vi "layout.vi"(0 "reference in":refnum<class "VINode.lvclass">, 1 "graph":refnum<class "Graph.lvclass">, 2 "graphics":refnum<class "Graphics.lvclass">, 3 "grid":refnum<class "Grid.lvclass">, 5 "error in (no error)":errorcluster) -> (14 "reference out":refnum<class "VINode.lvclass">, 19 "error out":errorcluster)   [LabVIEW 2020, in "VINode.lvclass"]
doc: "public void layout(Graph g, Graphics2D g2, Grid grid)"
uses:
  <resource>/Framework/Providers/Open_GDS/UML/VINode_class/VINode.lvclass
  C:/Program Files (x86)/National Instruments/LabVIEW 2020/resource/Framework/Providers/Open_GDS/UML/RectangularNode_class/RectangularNode.lvclass
  <resource>/Framework/Providers/Open_GDS/UML/Graph_class/Graph.lvclass
  <resource>/Framework/Providers/Open_GDS/UML/Graphics_class/Graphics.lvclass
  <resource>/Framework/Providers/Open_GDS/UML/Grid_class/Grid.lvclass
  <resource>/Framework/Providers/Open_GDS/UML/General/Rectangle/Rectangle Rectangle2D.ctl
  <resource>/Framework/Providers/Open_GDS/UML/MultiLineString_class/MultiLineString.lvclass
  <resource>/Framework/Providers/Open_GDS/UML/RectangularNode_class/RectangularNode.lvclass
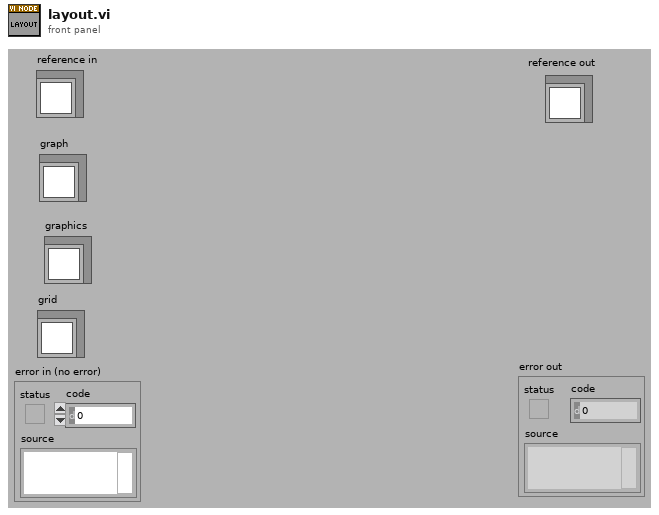
[diagram p1: front panel]
types:
  T1 = typedef "Rectangle Rectangle2D.ctl" = cluster{"x":dbl, "y":dbl, "width":dbl, "height":dbl}
  T2 = typedef "VINode.lvclass/ObjectAttributes.ctl" = cluster{"midHeight":dbl, "botHeight":dbl, "Name":refnum<class "MultiLineString.lvclass">, "DEFAULT_COMPARTMENT_HEIGHT":i32, "DEFAULT_WIDTH":i32, "DEFAULT_HEIGHT":i32, "VIPath":path, "Description":refnum<class "MultiLineString.lvclass">, "ShowDescription":bool}
  T3 = typedef "RectangularNode.lvclass/ObjectAttributes.ctl" = cluster{"bounds":T1}
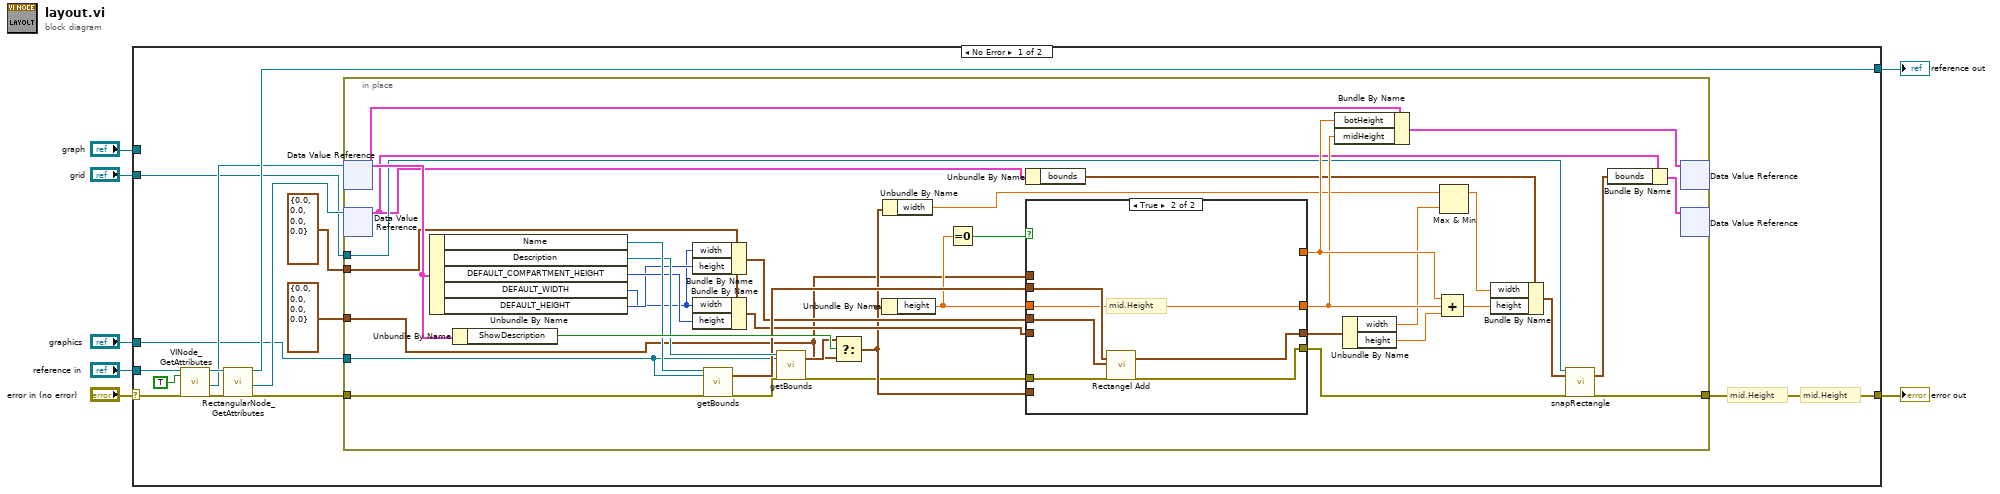
[diagram p0: block diagram]
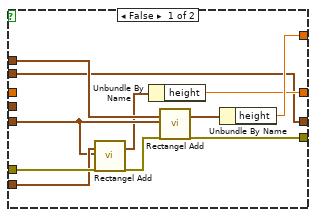
[diagram p2: hidden frame]
diagram:
  n1 = case shown="No Error" "error in (no error)" {
    selector: "error in (no error)" -> [w18 w76]
    tunnel: "reference in" -> [w21 w77]
    tunnel: [w20 w76] -> w6
    tunnel: [w19 w77] -> w5
    tunnel: "graph" -> [_ _]
    tunnel: "graphics" -> [w10 _]
    tunnel: "grid" -> [w8 _]
    frame No Error {
      # "mid.Height"
      # "mid.Height"
      n2 = call <resource>:"VINode_GetAttributes.vi"("reference in"=w21, "OnlyGetDvrReference(False)"=TRUE, "error in (no error)"=w18) -> ("reference out"=w16:refnum<class "VINode.lvclass">, "DataRef"=w14:refnum<data-value>, "error out"=w15:errorcluster)  [unwired: 13 in, 1 out]
      n3 = call <resource>:"RectangularNode_GetAttributes.vi"("reference in"=w16, "error in (no error)"=w15) -> ("reference out"=w19:refnum<class "VINode.lvclass">, "DataRef"=w13:refnum<data-value>, "error out"=w11:errorcluster)  [unwired: 14 in, 1 out]
      n4 = in-place {
        in-place-border: T1 {"x"=0.0, "y"=0.0, "width"=0.0, "height"=0.0} ("f") -> [w25]
        in-place-border: w11 -> [w39]
        in-place-border: w10 -> [w37]
        in-place-border: T1 {"x"=0.0, "y"=0.0, "width"=0.0, "height"=0.0} ("bounds") -> [w36]
        in-place-border: w8 -> [w35]
        in-place-border: [w32] -> w20
        n5 = in-place-dvr #1(w14) -> (w58:T2)  [unwired: 1 out]
        n6 = in-place-dvr #2(w13) -> (w28:T3)  [unwired: 1 out]
        n7 = Unbundle By Name(w58) -> ("Name"=w53:refnum<class "MultiLineString.lvclass">, "Description"=w52:refnum<class "MultiLineString.lvclass">, "DEFAULT_COMPARTMENT_HEIGHT"=w51:i32, "DEFAULT_WIDTH"=w22:i32, "DEFAULT_HEIGHT"=w50:i32)
        n8 = Unbundle By Name(w58) -> ("ShowDescription"=w54:bool)
        n9 = Bundle By Name(cluster=w36, "width"=w22, "height"=w50) -> (w48:T1)
        n10 = Bundle By Name(cluster=w36, "width"=w22, "height"=w51) -> (w47:T1)
        n11 = call-dynamic "getBounds.vi"("reference"=w53, "graphics"=w37, "error in (no error)"=w39) -> ("bounds"=w49:T1, "error out"=w38:errorcluster)  [unwired: 15 out]
        n12 = call-dynamic "getBounds.vi"("reference"=w52, "graphics"=w37, "error in (no error)"=w38) -> ("bounds"=w40:T1, "error out"=w26:errorcluster)  [unwired: 15 out]
        n13 = Select(t=w40, s=w54, f=w25) -> (s? t:f=w46:T1)
        n14 = Unbundle By Name(w46) -> ("height"=w45:dbl)
        n15 = Unbundle By Name(w46) -> ("width"=w23:dbl)
        n16 = Equal To 0?(x=w45) -> (x = 0?=w24:bool)
        n17 = Unbundle By Name(w28) -> ("bounds"=w30:T1)
        n18 = case shown="True" w24 {
          tunnel: w49 -> [w59 w75]
          tunnel: w48 -> [_ w74]
          tunnel: w26 -> [w69 w73]
          tunnel: w47 -> [w66 _]
          tunnel: w46 -> [w68 _]
          tunnel: w25 -> [w65 _]
          tunnel: [w62 _] -> w57
          tunnel: w45 -> [_ w72]
          tunnel: [w61 w72] -> w56
          tunnel: [w60 w71] -> w44
          tunnel: [w59 w70] -> w43
          frame False {
            n19 = call <resource>:"Rectangel Add.vi"("bounds1"=w68, "bounds2"=w66, "error in (no error)"=w69) -> ("boundsAdded"=w64:T1, "error out"=w67:errorcluster)  [unwired: 2 in, 13 out]
            n20 = Unbundle By Name(w64) -> ("height"=w61:dbl)
            n21 = call <resource>:"Rectangel Add.vi"("bounds1"=w65, "bounds2"=w66, "error in (no error)"=w67) -> ("boundsAdded"=w63:T1, "error out"=w60:errorcluster)  [unwired: 2 in, 13 out]
            n22 = Unbundle By Name(w63) -> ("height"=w62:dbl)
          }
          frame True {
            # "mid.Height"
            n23 = call <resource>:"Rectangel Add.vi"("bounds1"=w75, "bounds2"=w74, "error in (no error)"=w73) -> ("boundsAdded"=w70:T1, "error out"=w71:errorcluster)  [unwired: 2 in, 13 out]
          }
        }
        n24 = Bundle By Name(cluster=w58, "botHeight"=w57, "midHeight"=w56) -> (w55:T2)
        n25 = Unbundle By Name(w43) -> ("width"=w31:dbl, "height"=w42:dbl)
        n26 = Max & Min(x=w23, y=w31) -> (max(x,y)=w29:dbl)  [unwired: 1 out]
        n27 = Compound Arithmetic op=ADD(w57, w56, w42) -> (w41:dbl)
        n28 = Bundle By Name(cluster=w30, "width"=w29, "height"=w41) -> (w34:T1)
        n29 = call <resource>:"snapRectangle.vi"("reference"=w35, "bounds"=w34, "error in (no error)"=w44) -> ("boundsOut"=w33:T1, "error out"=w32:errorcluster)  [unwired: 15 out]
        n30 = Bundle By Name(cluster=w28, "bounds"=w33) -> (w27:T3)
        n31 = in-place-dvr #1(w55) -> ()  [unwired: 2 out]
        n32 = in-place-dvr #2(w27) -> ()  [unwired: 2 out]
      }
    }
    frame Error {
    }
  }
  "reference out" <- w5
  "error out" <- w6
